vi "String to Character Array.vi"(1 "input string":string="\n\r\t") -> (0 "character array":string[](array[string]))   [LabVIEW 2020]
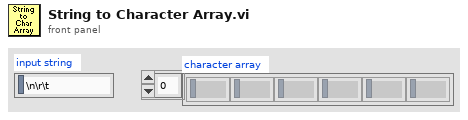
[diagram p1: front panel]
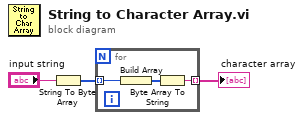
[diagram p0: block diagram]
diagram:
  n1 = String To Byte Array(string="input string") -> (unsigned byte array=w2:u8[])
  n2 = for {
    tunnel: w2 -> [w6] mode=indexing
    tunnel: [w4] -> w1 mode=indexing
    n3 = Build Array(w6) -> (w5:u8[])
    n4 = Byte Array To String(unsigned byte array=w5) -> (string=w4:string)
  }
  "character array" <- w1
